vi "event_duration.vi"(7 "wavelet array length":i32, 10 "Input Outlier indices":T1) -> (0 "t_c":dbl[](array[numeric]), 1 "t_b":dbl[](array[numeric]), 2 "t_a":dbl[](array[numeric]))   [LabVIEW 2014]
uses:
  <vilib>/imath/engines/lvmath2/RunTimeEngine/BuiltInFunctions/is_empty/NIMS_is_empty(GV).vi
  <instcachedir>/0/NIMS_is_empty(GV)_FC7E7C3D9544432CB6AA2416ADCF6D56.lvgen/NIMS_is_empty(GV)_FC7E7C3D9544432CB6AA2416ADCF6D56_000.vi
  <vilib>/imath/engines/lvmath2/RunTimeEngine/BuiltInFunctions/difference/NIMS_difference(GV,I32).vi
  <instcachedir>/0/NIMS_difference(GV,I32)_DC7351DCBCF840A8AE147F50EC2CE86E.lvgen/NIMS_difference(GV,I32)_DC7351DCBCF840A8AE147F50EC2CE86E_000.vi
  <vilib>/imath/engines/lvmath2/RunTimeEngine/BuiltInFunctions/findnz/NIMS_[1o]_findnz(GRowV).vi
  <instcachedir>/0/NIMS_[1o]_findnz(GRowV)_09DEEFCD766A4095B33095726AFD3FF8.lvgen/NIMS_[1o]_findnz(GRowV)_09DEEFCD766A4095B33095726AFD3FF8_000.vi
  <vilib>/imath/engines/lvmath2/RunTimeEngine/IndexRead/NIMS V(S).vi
  <instcachedir>/0/NIMS V(S)_0488751826AF41519A22953C041130DC.lvgen/NIMS V(S)_0488751826AF41519A22953C041130DC_002.vi
  <vilib>/imath/engines/lvmath2/RunTimeEngine/IndexRead/NIMS V(V).vi
  <instcachedir>/0/NIMS V(V)_298D9CB7BFEB42B8BC8D9C3C28AE8C70.lvgen/NIMS V(V)_298D9CB7BFEB42B8BC8D9C3C28AE8C70_001.vi
  <vilib>/imath/engines/lvmath2/RunTimeEngine/ErrorHandling/NIMS_Create Error From Enums.vi
  <vilib>/imath/engines/lvmath2/RunTimeEngine/BuiltInFunctions/linramp/NIMS_linramp.vi
  <vilib>/imath/engines/lvmath2/RunTimeEngine/IndexRead/NIMS V(M).vi
  <instcachedir>/0/NIMS V(M)_9C733378D59448EDB8B370EA0429D12A.lvgen/NIMS V(M)_9C733378D59448EDB8B370EA0429D12A_000.vi
  <vilib>/imath/engines/lvmath2/RunTimeEngine/ArithmeticOperatorToken/NIMS_ArithmeticOperator_minus.vi
  <instcachedir>/0/NIMS_ArithmeticOperator_minus_39C0593E74DA4138ACA2AB742906488D.lvgen/NIMS_ArithmeticOperator_minus_39C0593E74DA4138ACA2AB742906488D_002.vi
  <vilib>/imath/engines/lvmath2/RunTimeEngine/NodeEndStatement/NIMS_NodeEndStatement_Get Vector.vi
  <instcachedir>/0/NIMS_NodeEndStatement_Get Vector_00D1625602D843AD9D7EC134A9EC13A2.lvgen/NIMS_NodeEndStatement_Get Vector_00D1625602D843AD9D7EC134A9EC13A2_001.vi
  <vilib>/imath/engines/lvmath/Functions/Error Handling/MergeErrorsWrapper.vi
  <vilib>/imath/engines/lvmath2/RunTimeEngine/NodeEndStatement/NIMS_NodeEndStatement_Output.vi
  <instcachedir>/0/NIMS_NodeEndStatement_Output_53EC0D466D134D7ABD903AC30B43404B.lvgen/NIMS_NodeEndStatement_Output_53EC0D466D134D7ABD903AC30B43404B_005.vi
  <vilib>/imath/engines/lvmath2/RunTimeEngine/ErrorHandling/NIMS_Finalize Error.vi
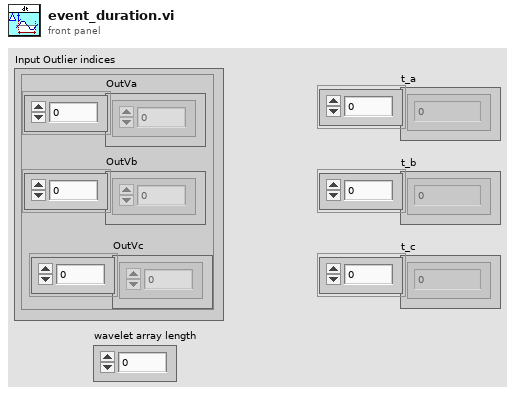
[diagram p1: front panel]
types:
  T1 = cluster{"OutVa":i32[], "OutVb":i32[], "OutVc":i32[]}
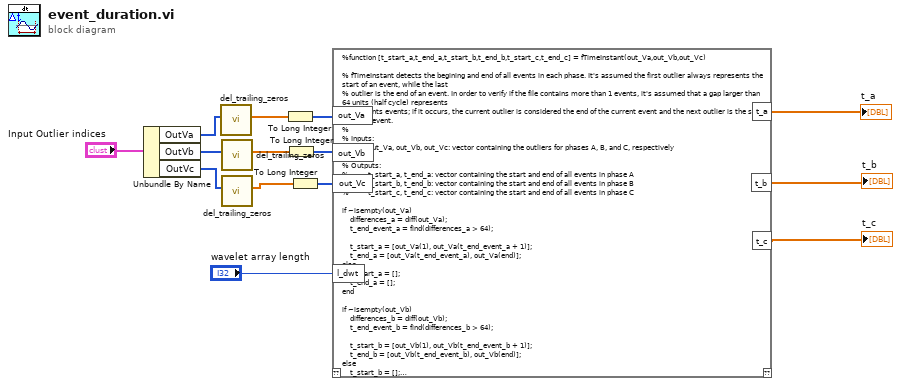
[diagram p0: block diagram]
diagram:
  n1 = Unbundle By Name("Input Outlier indices") -> ("OutVa"=w9:i32[], "OutVb"=w7:i32[], "OutVc"=w5:i32[])
  n2 = call "del_trailing_zeros.vi"("Array"=w9) -> ("Shortened array"=w8:dbl[])  [unwired: 10 in]
  n3 = call "del_trailing_zeros.vi"("Array"=w7) -> ("Shortened array"=w6:dbl[])  [unwired: 10 in]
  n4 = call "del_trailing_zeros.vi"("Array"=w5) -> ("Shortened array"=w4:dbl[])  [unwired: 10 in]
  n5 = To Long Integer(number=w8) -> (32bit integer=w3:i32[])
  n6 = To Long Integer(number=w6) -> (32bit integer=w2:i32[])
  n7 = To Long Integer(number=w4) -> (32bit integer=w1:i32[])
  n8 = mathscript code="%function [t_start_a,t_end_a,t_start_b,t_end_b,t_start_c,t_end_c] = fTimeInstant(out_Va,out_Vb,out_Vc)\n\n% fTimeInstant detects the begining and end of all events in each phase. It's assumed the first outlier always represents the start of an event, while the last\n% outlier is the end of an event. In order to verify if the file contains more than 1 events, it's assumed that a gap larger than 64 units (half cycle) represents\n% differents events; if it occurs, the current outlier is considered the end of the current event and the next outlier is the start of a new event.\n%\n% Inputs:\n%       - out_Va, out_Vb, out_Vc: vector containing the outliers for phases A, B, and C, respectively\n%\n% Outputs:\n%       - t_start_a, t_end_a: vector containing the start and end of all events in phase A\n%       - t_start_b, t_end_b: vector containing the start and end of all events in phase B\n%       - t_start_c, t_end_c: vector containing the start and end of all events in phase C\n\nif ~isempty(out_Va)\n    differences_a = diff(out_Va);\n    t_end_event_a = find(differences_a > 64); \n\n    t_start_a = [out_Va(1), out_Va(t_end_event_a + 1)];\n    t_end_a = [out_Va(t_end_event_a), out_Va(end)];\nelse\n    t_start_a = [];\n    t_end_a = [];\nend\n\nif ~isempty(out_Vb)\n    differences_b = diff(out_Vb);\n    t_end_event_b = find(differences_b > 64); \n\n    t_start_b = [out_Vb(1), out_Vb(t_end_event_b + 1)];\n    t_end_b = [out_Vb(t_end_event_b), out_Vb(end)];\nelse\n    t_start_b = [];\n    t_end_b = [];\nend\n\nif ~isempty(out_Vc)\n    differences_c = diff(out_Vc);\n    t_end_event_c = find(differences_c > 64); \n\n    t_start_c = [out_Vc(1), out_Vc(t_end_event_c + 1)];\n    t_end_c = [out_Vc(t_end_event_c), out_Vc(end)];\nelse\n    t_start_c = [];\n    t_end_c = [];\nend\n% Transform indices from wavelet scale to time\nt_wav = linspace(0,30,l_dwt);\n    \n% Duration (in seconds)\nt_a = t_wav(t_end_a) - t_wav(t_start_a);\nt_b = t_wav(t_end_b) - t_wav(t_start_b); \nt_c = t_wav(t_end_c) - t_wav(t_start_c);"("out_Va"=w3, "out_Vb"=w2, "out_Vc"=w1, "l_dwt"="wavelet array length") -> ("t_a"=→"t_a":dbl[], "t_b"=→"t_b":dbl[], "t_c"=→"t_c":dbl[])  [unwired: 1 in, 1 out]
